vi "CIMAQ_Create_Grayscale_UID.vi"   [LabVIEW 2017]
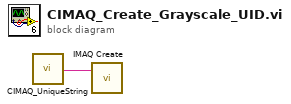
[diagram p0: block diagram]
diagram:
  n1 = call <userlib>:"CIMAQ_UniqueString.vi"() -> ("String"=w1:string)  [unwired: 5 in]
  n2 = call "IMAQ Create"("Image Name"=w1) -> ()  [unwired: 4 in, 2 out]
